vi "getFPGA.vi"(11 "HealthAndStatusDataFIFO in":refnum<class "HealthAndStatusDataFIFO.lvclass">) -> (2 "FPGA":refnum<class "FPGA.lvclass">, 3 "HealthAndStatusDataFIFO out":refnum<class "HealthAndStatusDataFIFO.lvclass">)   [LabVIEW 2016, in "HealthAndStatusDataFIFO.lvclass"]
uses:
  HealthAndStatusDataFIFO.lvclass
  FPGA/FPGA.lvclass
  HealthAndStatusDataFIFO.lvclass/HealthAndStatusDataFIFO.ctl
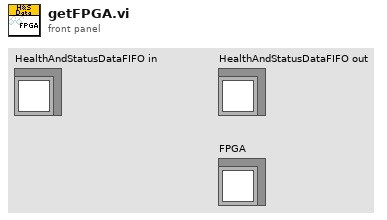
[diagram p1: front panel]
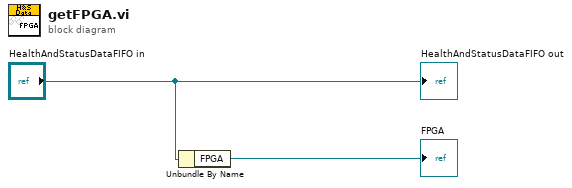
[diagram p0: block diagram]
diagram:
  n1 = Unbundle By Name("HealthAndStatusDataFIFO in") -> ("FPGA"=→"FPGA":refnum<class "FPGA.lvclass">)
  "HealthAndStatusDataFIFO out" <- "HealthAndStatusDataFIFO in"
